vi "Global_CMD to SM Data.vi"() -> ()   [LabVIEW 2017, in "Hopper System.lvlib"]
uses:
  Systems/Hopper/Hopper System.lvlib
  Systems/Hopper/Cluster_CMD to SM Data.ctl
  Systems/Hopper/ENUM_Firing_State.ctl
panel:
  out "Hopper Stop_CMD":bool
  in  "Inner Motor Speed_CMD":dbl=0.4
  in  "Loader Speed_CMD":dbl=0.4
  out "Hopper_CMD":T1={"Enable Loading"=FALSE, "Disable Loading"=FALSE, "Fireing State"=enum."No Fireing", "Time Limit Loading"=5.0, "Time Limit Rapid"=2.0, "Rapid Fire Shot Limit"=3, "Shotgun Fire Shot Limit"=1}
  # "WHEN CODE IS MERGED\nMOVE TO GLOBALS IN MAIN CODE\nOUTSIDE OF LIBRARY"
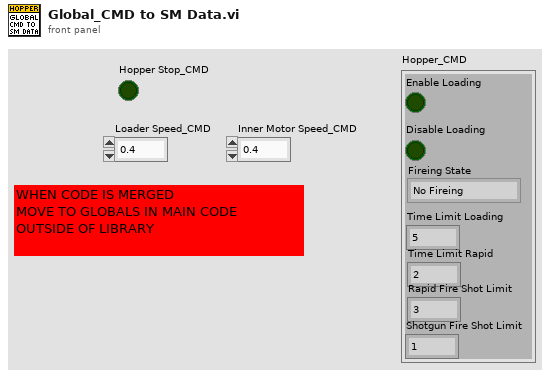
[diagram p1: front panel]
types:
  T1 = typedef "Hopper System.lvlib/Cluster_CMD to SM Data.ctl" = cluster{"Enable Loading":bool, "Disable Loading":bool, "Fireing State":T2, "Time Limit Loading":dbl, "Time Limit Rapid":dbl, "Rapid Fire Shot Limit":i32, "Shotgun Fire Shot Limit":i32}
  T2 = typedef "Hopper System.lvlib/ENUM_Firing_State.ctl" = enum16{"No Fireing", "Rapid Fire", "Shotgun Fireing"}
diagram:
